vi "20151112 condition.vi"(4 "Condition":T2, 5 "State":T1) -> (2 "result":bool)   [LabVIEW 2013]
uses:
  Q-neural/controls/Sample set.ctl
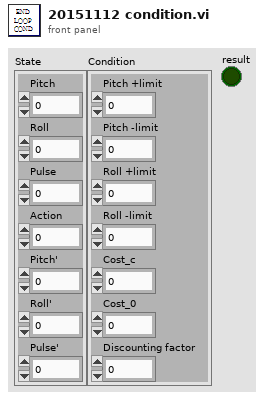
[diagram p1: front panel]
types:
  T1 = typedef "Sample set.ctl" = cluster{"Pitch":dbl, "Roll":dbl, "Pulse":dbl, "Action":dbl, "Pitch'":dbl, "Roll'":dbl, "Pulse'":dbl}
  T2 = cluster{"Pitch +limit":dbl, "Pitch -limit":dbl, "Roll +limit":dbl, "Roll -limit":dbl, "Cost_c":dbl, "Cost_0":dbl, "Discounting factor":dbl}
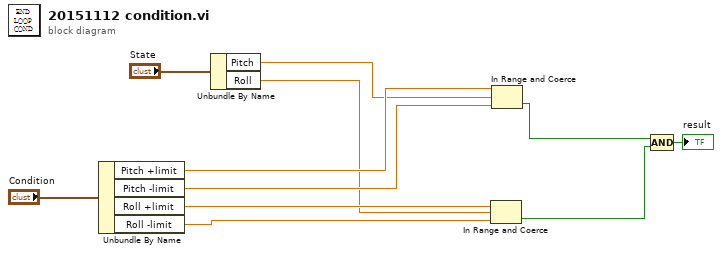
[diagram p0: block diagram]
diagram:
  n1 = Unbundle By Name("Condition") -> ("Pitch +limit"=w8:dbl, "Pitch -limit"=w9:dbl, "Roll +limit"=w10:dbl, "Roll -limit"=w11:dbl)
  n2 = Unbundle By Name("State") -> ("Pitch"=w4:dbl, "Roll"=w5:dbl)
  n3 = In Range and Coerce(upper limit=w10, x=w5, lower limit=w11) -> (In Range?=w7:bool)  [unwired: 1 out]
  n4 = In Range and Coerce(upper limit=w8, x=w4, lower limit=w9) -> (In Range?=w6:bool)  [unwired: 1 out]
  n5 = Compound Arithmetic op=AND(w6, w7) -> (→"result":bool)
